vi "Write Pulse Generator.lvclass.vi"(8 "error in (no error)":errorcluster, 10 "Pulse Generator.lvclass":refnum<class "Pulse Generator.lvclass">=refnum, 11 "SPARC4_AC in":refnum<class "S4ACS_GUI.lvclass">) -> (0 "error out":errorcluster, 3 "SPARC4_AC out":refnum<class "S4ACS_GUI.lvclass">)   [LabVIEW 2012, in "S4ACS_GUI.lvclass"]
uses:
  S4ACS_GUI.lvclass
  SPARC4 - 12-11-2020/SPARC4 GUI test/SPARC4/SPARC4_GUI/Pulse Generator/Pulse Generator.lvclass
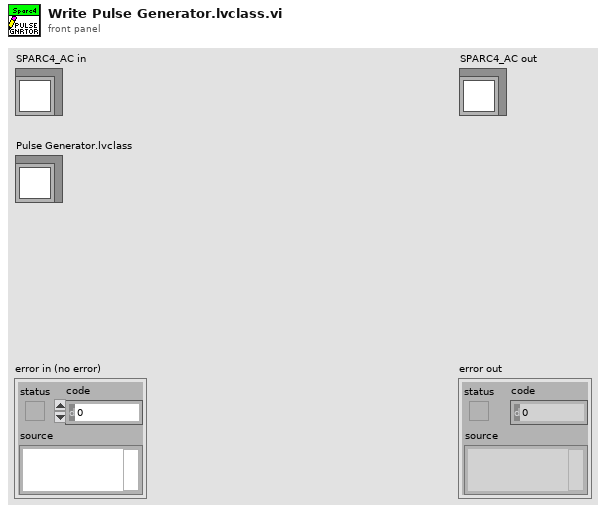
[diagram p1: front panel]
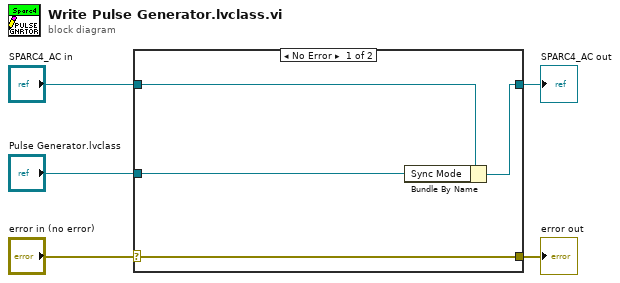
[diagram p0: block diagram]
diagram:
  n1 = case shown="No Error" "error in (no error)" {
    selector: "error in (no error)" -> [w9 w10]
    tunnel: [w9 w10] -> w4
    tunnel: [w7 w11] -> w2
    tunnel: "SPARC4_AC in" -> [w8 w11]
    tunnel: "Pulse Generator.lvclass" -> [w6 _]
    frame No Error {
      n2 = Bundle By Name(cluster=w8, "Sync Mode"=w6) -> (w7:refnum<class "S4ACS_GUI.lvclass">)
    }
    frame Error {
    }
  }
  "error out" <- w4
  "SPARC4_AC out" <- w2
